vi "全局 数据数组大小.vi"() -> ()   [LabVIEW 2016]
panel:
  out "数据数组大小":i32
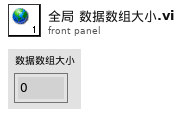
[diagram p1: front panel]
diagram:
